vi "eventlog parse GET.vi"(7 "GET (empty)":T1) -> (2 "parameter":string, 3 "Command":string)   [LabVIEW 2011]
uses:
  Addons/internet/utils/keyedarr.llb/Keyed Array.ctl
  Addons/internet/utils/strutil.llb/Case Matching.ctl
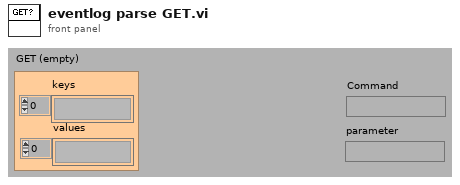
[diagram p1: front panel]
types:
  T1 = typedef "Keyed Array.ctl" = cluster{"keys":string[], "values":string[]}
  T2 = typedef "Case Matching.ctl" = enum16{"a != A", "a == A", "system"}
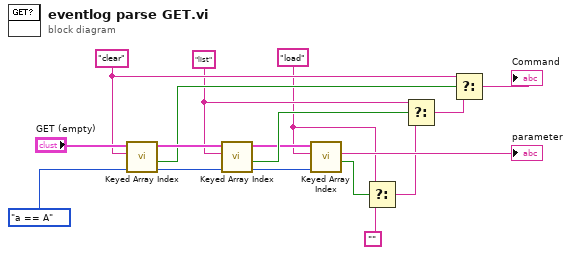
[diagram p0: block diagram]
diagram:
  w2 = "load" ("Template (\"\")")
  w6 = Case_Matching."a == A" ("case matching (sensitive)")
  w12 = "clear" ("Template (\"\")")
  w10 = "list" ("Template (\"\")")
  n1 = call "Keyed Array Index.vi"("case matching (sensitive)"=w6, "key"=w12, "array in"="GET (empty)") -> ("valid key"=w13:bool, "duplicate array"=w14:T1)  [unwired: 1 in, 2 out]
  n2 = call "Keyed Array Index.vi"("case matching (sensitive)"=w6, "key"=w10, "array in"=w14) -> ("valid key"=w9:bool, "duplicate array"=w7:T1)  [unwired: 1 in, 2 out]
  n3 = call "Keyed Array Index.vi"("case matching (sensitive)"=w6, "key"=w2, "array in"=w7) -> ("valid key"=w3:bool, "value"=→"parameter":string)  [unwired: 1 in, 2 out]
  n4 = Select(t=w2, s=w3, f="") -> (s? t:f=w1:string)
  n5 = Select(t=w10, s=w9, f=w1) -> (s? t:f=w8:string)
  n6 = Select(t=w12, s=w13, f=w8) -> (s? t:f=→"Command":string)
